vi "[Debug] Global.vi"() -> ()   [LabVIEW 2009]
panel:
  out "DD Error":fxp<+/-,18,1> format="%.18g"
  out "DD portion":fxp<+/-,18,1> format="%.18g"
  out "D Error":fxp<+/-,18,1> format="%.18g"
  out "II Error":fxp<+/-,18,1> format="%.18g"
  out "I Error":fxp<+/-,18,1> format="%.18g"
  out "P Error":fxp<+/-,18,1> format="%.18g"
  out "D portion":fxp<+/-,18,1> format="%.18g"
  out "II portion":fxp<+/-,18,1> format="%.18g"
  out "I portion":fxp<+/-,18,1> format="%.18g"
  out "P portion":fxp<+/-,18,1> format="%.18g"
  out "Server 1 Timeouts by Identifier":bool[](array[boolean])
  out "p gain":fxp<+/-,18,1> format="%.18g"
  out "pregain":fxp<+/-,18,1> format="%.18g"
  out "after 5th":fxp<+/-,18,1> format="%.18g"
  out "after 4th":fxp<+/-,18,1> format="%.18g"
  out "After 3rd":fxp<+/-,18,1> format="%.18g"
  out "After Second Multiply":fxp<+/-,18,1> format="%.18g"
  out "After first multiply":fxp<+/-,18,1> format="%.18g"
  out "Error in Fxp 18b":fxp<+/-,18,1> format="%.18g"
  out "Lidar setpoint 32b int (enc)":i32
  out "Error 32b int (enc)":i32
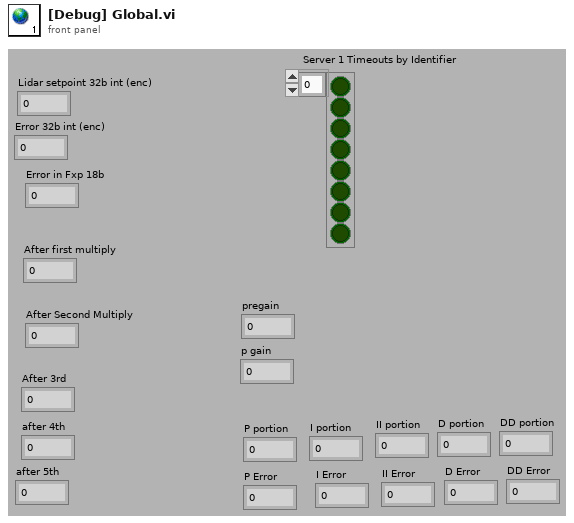
[diagram p1: front panel]
diagram:
